vi "main.vi"() -> ()   [LabVIEW 2023]
panel:
  in  "Pause Game":bool
  in  "Decrease\nPlayer Length":bool
  in  "Stop":bool
  out "p2 score":i32
  out "p1 score":i32
  in  "w_bool":bool
  in  "Down_bool":bool
  in  "s_bool":bool
  in  "Up_bool":bool
  out "game window":picture
  # "Player 1: W, S\nPlayer 2: Up, Down"
  # "Modifiers"
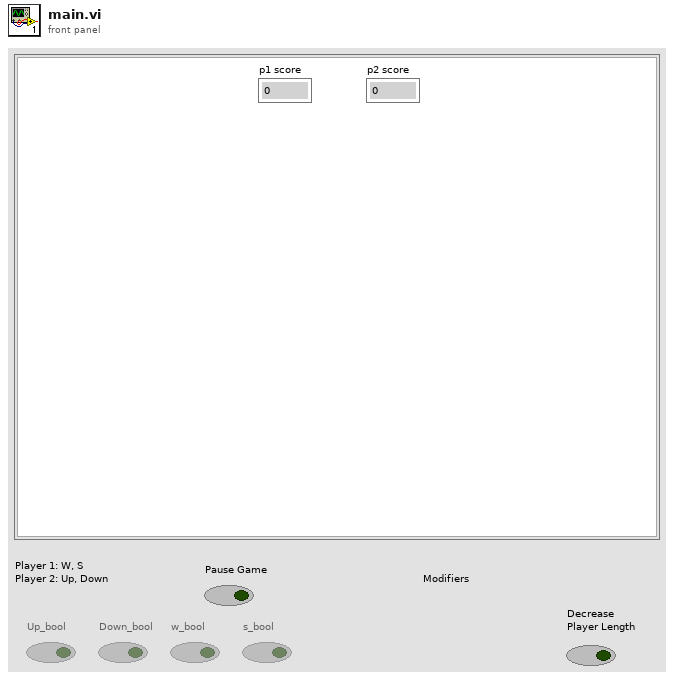
[diagram p1: front panel]
types:
  T1 = cluster{"output vector x":dbl, "output vector y":dbl}
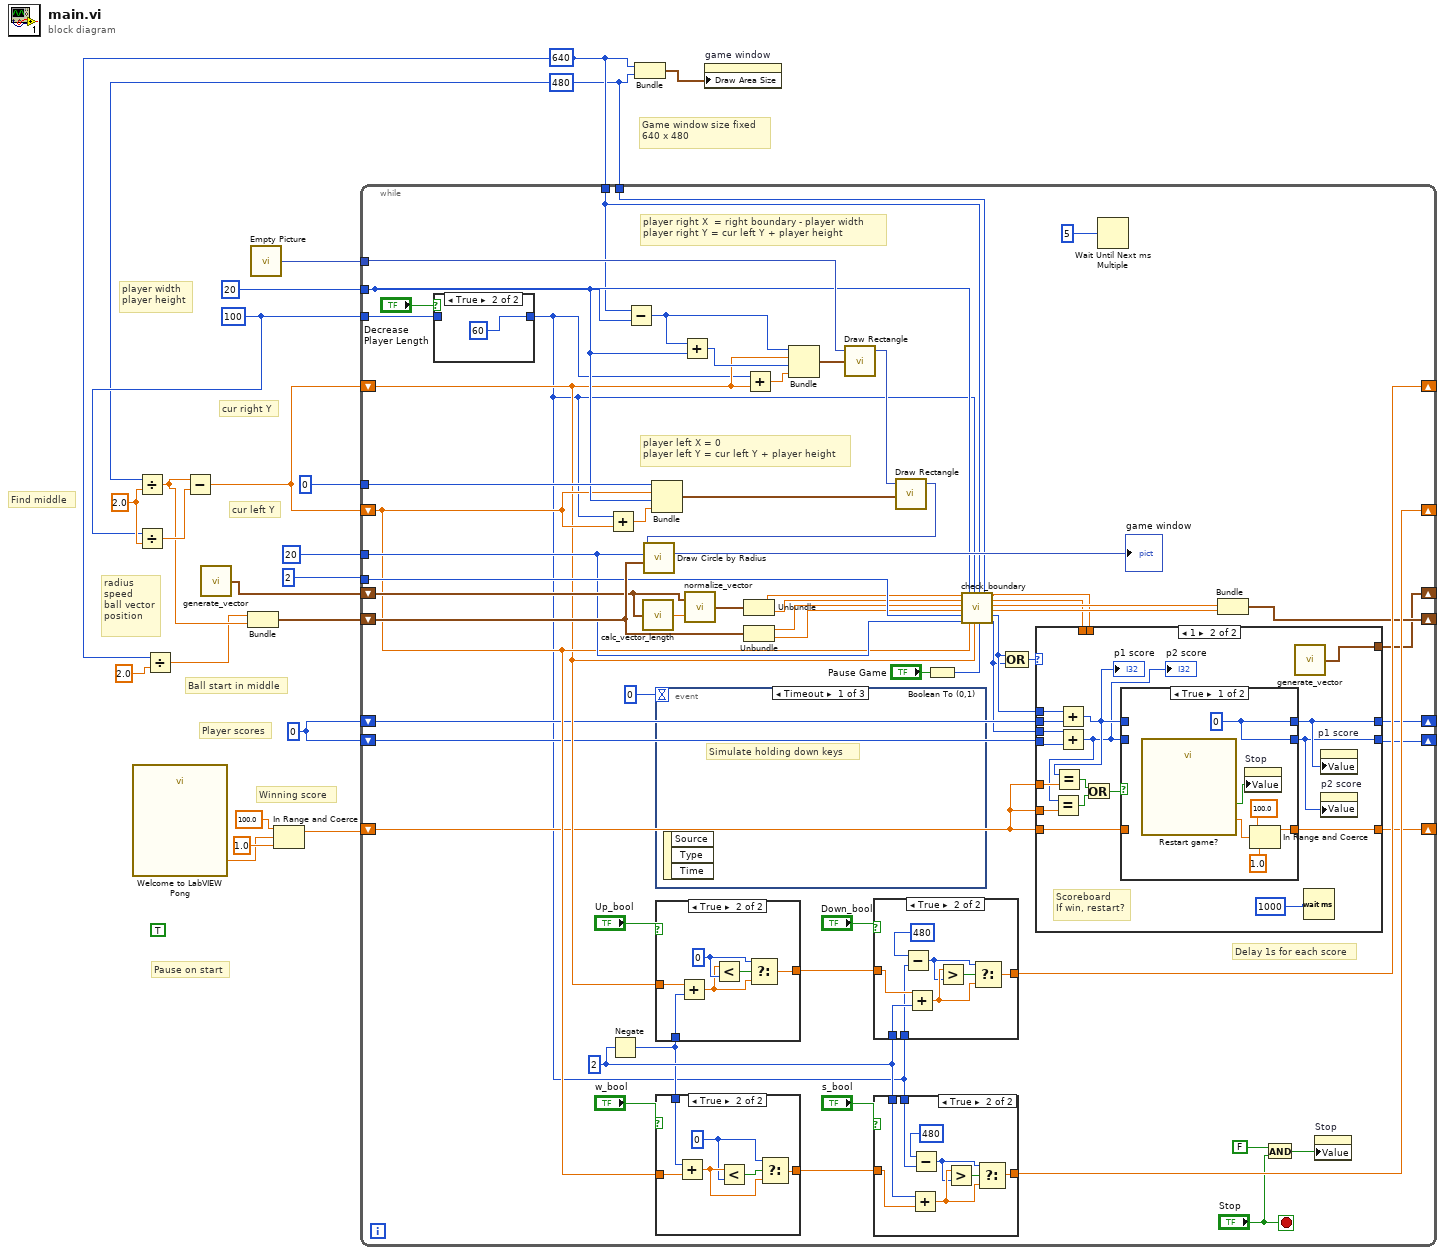
[diagram p0: block diagram]
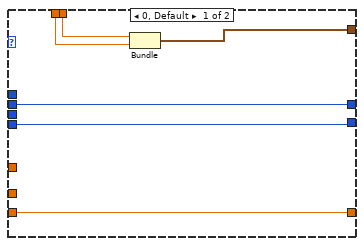
[diagram p3: hidden frame]
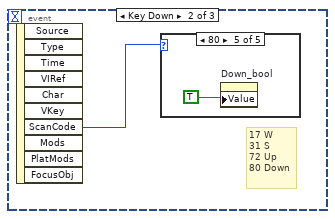
[diagram p9: hidden frame]
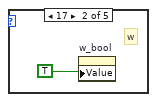
[diagram p11: hidden frame]
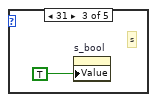
[diagram p12: hidden frame]
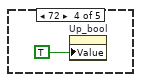
[diagram p13: hidden frame]
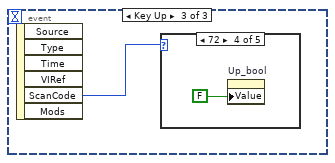
[diagram p14: hidden frame]
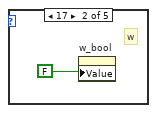
[diagram p16: hidden frame]
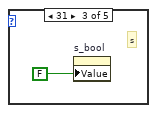
[diagram p17: hidden frame]
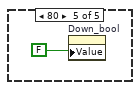
[diagram p18: hidden frame]
diagram:
  (unwired) TRUE ("Pause Game")
  w6 = 0
  w7 = 480
  w14 = 640
  w17 = 2.0 ("y")
  w15 = 100
  # "Pause on start"
  # "Winning score"
  # "Player scores"
  # "Ball start in middle"
  # "radius\nspeed\nball vector\nposition"
  # "Find middle"
  # "player width\nplayer height"
  # "cur left Y"
  # "cur right Y"
  # "Game window size fixed\n640 x 480"
  n1 = call "Welcome to LabVIEW Pong"() -> ("Winning Score"=w2:dbl)  [unwired: 17 in, 2 out]
  n2 = Divide(x=w7, y=w17) -> (x/y=w11:dbl)
  n3 = Divide(x=w15, y=w17) -> (x/y=w16:dbl)
  n4 = Divide(x=w14, y=2.0) -> (x/y=w10:dbl)
  n5 = Subtract(x=w11, y=w16) -> (x-y=w18:dbl)
  n6 = call "generate_vector.vi"() -> ("Cluster"=w5:cluster{"number":dbl, "number":dbl})
  n7 = Bundle(w10, w11) -> (w12:cluster{dbl, dbl})  [unwired: 1 in]
  n8 = call "Empty Picture"() -> ("empty picture"=w21:picture)
  n9 = In Range and Coerce(upper limit=100.0, x=w2, lower limit=1.0) -> (coerced(x)=w3:dbl)  [unwired: 1 out]
  n10 = while {
    tunnel: w14 -> [w50]
    tunnel: w21 -> [w80]
    shift-right: [w68] -> _
    shift-left: w18 -> [w43]
    shift-right: [w66] -> _
    shift-left: w18 -> [w44]
    tunnel: w15 -> [w27]
    tunnel: 20 -> [w51]
    tunnel: 0 -> [w78]
    shift-right: [w35] -> _
    shift-left: w5 -> [w57]
    shift-right: [w46] -> _
    shift-left: w12 -> [w60]
    tunnel: 20 -> [w45]
    tunnel: 2 -> [w56]
    tunnel: w7 -> [w49]
    shift-right: [w42] -> _
    shift-left: w6 -> [w40]
    shift-right: [w41] -> _
    shift-left: w6 -> [w39]
    shift-right: [w38] -> _
    shift-left: w3 -> [w31]
    stop <- "Stop" stop-if-true
    w71 = 2 ("y")
    # "Delay 1s for each score"
    # "player right X  = right boundary - player width\nplayer right Y = cur left Y + player height"
    # "player left X = 0\nplayer left Y = cur left Y + player height"
    n11 = case shown="True" "Decrease\nPlayer Length" {
      tunnel: w27 -> [w84 _]
      tunnel: [w84 60] -> w26
      frame False {
      }
      frame True {
      }
    }
    n12 = Add(x=w26, y=w44) -> (x+y=w77:dbl)
    n13 = Negate(x=w71) -> (-x=w70:i32)
    n14 = Subtract(x=w50, y=w51) -> (x-y=w83:i32)
    n15 = call "calc_vector_length.vi"("vector"=w57) -> ("length"=w58:dbl)
    n16 = Bundle(w78, w44, w51, w77) -> (w76:cluster{i32, dbl, i32, dbl})  [unwired: 1 in]
    n17 = event shown="[0] Timeout" {
      selector: _ -> [_ _ _]
      dyn-events: _ -> [_ _ _]
      timeout: 0 -> [_ _ _]
      event Timeout {
        # "Simulate holding down keys"
        n18 = event-data() -> ()  [unwired: 1 in, 3 out]
      }
      event Key Down {
        # "17 W\n31 S\n72 Up\n80 Down"
        n19 = event-data() -> ("ScanCode"=w150:i16)  [unwired: 1 in, 9 out]
        n20 = case shown="80" w150 {
          frame 0, Default {
          }
          frame 17 {
            # "w"
            n21 = property on="w_bool" class="Bool (strict)"("Value"=TRUE) -> ()  [unwired: 2 in, 2 out]
          }
          frame 31 {
            # "s"
            n22 = property on="s_bool" class="Bool (strict)"("Value"=TRUE) -> ()  [unwired: 2 in, 2 out]
          }
          frame 72 {
            n23 = property on="Up_bool" class="Bool (strict)"("Value"=TRUE) -> ()  [unwired: 2 in, 2 out]
          }
          frame 80 {
            n24 = property on="Down_bool" class="Bool (strict)"("Value"=TRUE) -> ()  [unwired: 2 in, 2 out]
          }
        }
      }
      event Key Up {
        n25 = event-data() -> ("ScanCode"=w155:i16)  [unwired: 1 in, 5 out]
        n26 = case shown="72" w155 {
          frame 0, Default {
          }
          frame 17 {
            # "w"
            n27 = property on="w_bool" class="Bool (strict)"("Value"=FALSE) -> ()  [unwired: 2 in, 2 out]
          }
          frame 31 {
            # "s"
            n28 = property on="s_bool" class="Bool (strict)"("Value"=FALSE) -> ()  [unwired: 2 in, 2 out]
          }
          frame 72 {
            n29 = property on="Up_bool" class="Bool (strict)"("Value"=FALSE) -> ()  [unwired: 2 in, 2 out]
          }
          frame 80 {
            n30 = property on="Down_bool" class="Bool (strict)"("Value"=FALSE) -> ()  [unwired: 2 in, 2 out]
          }
        }
      }
    }
    n31 = case shown="True" "Up_bool" {
      tunnel: w70 -> [_ w145]
      tunnel: w43 -> [w143 w146]
      tunnel: [w143 w144] -> w69
      frame False {
      }
      frame True {
        w148 = 0 ("y")
        n32 = Add(x=w146, y=w145) -> (x+y=w147:dbl)
        n33 = Less?(x=w147, y=w148) -> (x < y?=w149:bool)
        n34 = Select(t=w148, s=w149, f=w147) -> (s? t:f=w144:dbl)
      }
    }
    n35 = case shown="True" "w_bool" {
      tunnel: w44 -> [w136 w138]
      tunnel: w70 -> [_ w139]
      tunnel: [w136 w137] -> w67
      frame False {
      }
      frame True {
        w140 = 0 ("y")
        n36 = Add(x=w139, y=w138) -> (x+y=w142:dbl)
        n37 = Less?(x=w142, y=w140) -> (x < y?=w141:bool)
        n38 = Select(t=w140, s=w141, f=w142) -> (s? t:f=w137:dbl)
      }
    }
    n39 = Add(x=w83, y=w51) -> (x+y=w82:i32)
    n40 = call "normalize_vector.vi"("Numeric"=w58, "vector"=w57) -> ("output"=w59:cluster{"x":dbl, "y":dbl})
    n41 = Unbundle(w59) -> ("x"=w55:dbl, "y"=w54:dbl)
    n42 = Unbundle(w60) -> (w53:dbl, w52:dbl)
    n43 = Add(x=w26, y=w43) -> (x+y=w81:dbl)
    n44 = Bundle(w83, w43, w82, w81) -> (w79:cluster{i32, dbl, i32, dbl})  [unwired: 1 in]
    n45 = call <vilib>:"Draw Rectangle.vi"("picture"=w80, "rect"=w79) -> ("new picture"=w75:picture)  [unwired: 7 in]
    n46 = case shown="True" "Down_bool" {
      tunnel: w71 -> [_ w131]
      tunnel: w69 -> [w127 w130]
      tunnel: [w127 w129] -> w68
      tunnel: w26 -> [_ w128]
      frame False {
      }
      frame True {
        n47 = Subtract(x=480 ("y"), y=w128) -> (x-y=w133:i32)
        n48 = Add(x=w130, y=w131) -> (x+y=w134:dbl)
        n49 = Greater?(x=w134, y=w133) -> (0:w135:bool)
        n50 = Select(t=w133, s=w135, f=w134) -> (s? t:f=w129:dbl)
      }
    }
    n51 = case shown="True" "s_bool" {
      tunnel: w71 -> [_ w121]
      tunnel: w67 -> [w118 w122]
      tunnel: [w118 w120] -> w66
      tunnel: w26 -> [_ w119]
      frame False {
      }
      frame True {
        n52 = Add(x=w121, y=w122) -> (x+y=w125:dbl)
        n53 = Subtract(x=480 ("y"), y=w119) -> (x-y=w124:i32)
        n54 = Greater?(x=w125, y=w124) -> (0:w126:bool)
        n55 = Select(t=w124, s=w126, f=w125) -> (s? t:f=w120:dbl)
      }
    }
    n56 = call <vilib>:"Draw Rectangle.vi"("picture"=w75, "rect"=w76) -> ("new picture"=w62:picture)  [unwired: 7 in]
    n57 = call <vilib>:"Draw Circle by Radius.vi"("pixel center"=w60, "radius"=w45, "picture"=w62) -> ("new picture"=→"game window":picture)  [unwired: 8 in]
    n58 = Boolean To (0,1)(Boolean="Pause Game") -> (0, 1=w23:i16)
    n59 = call "check_boundary.vi"("vector x"=w55, "vector y"=w54, "position x"=w53, "position y"=w52, "speed"=w56, "radius"=w45, "player width"=w51, "player left position y"=w44, "player height"=w26, "player right position y"=w43, "window width"=w50, "pause"=w23, "window height"=w49) -> ("output vector x"=w37:dbl, "output vector y"=w36:dbl, "output x"=w48:dbl, "output y"=w47:dbl, "left win"=w29:i32, "right win"=w28:i32)  [unwired: 1 in]
    n60 = Compound Arithmetic op=OR(w29, w28) -> (w30:i32)
    n61 = case shown="1" w30 {
      tunnel: w40 -> [w91 w99]
      tunnel: w39 -> [w90 w97]
      tunnel: w29 -> [_ w100]
      tunnel: w28 -> [_ w98]
      tunnel: [w91 w93] -> w42
      tunnel: [w90 w92] -> w41
      tunnel: w31 -> [_ w108]
      tunnel: w31 -> [_ w107]
      tunnel: [w89 w103] -> w38
      tunnel: w31 -> [w89 w102]
      tunnel: w37 -> [w88 _]
      tunnel: w36 -> [w87 _]
      tunnel: [w86 w101] -> w35
      frame 0, Default {
        n62 = Bundle("output vector x"=w88, "output vector y"=w87) -> (w86:T1)  [unwired: 1 in]
      }
      frame 1 {
        # "Scoreboard\nIf win, restart?"
        n63 = Add(x=w100, y=w99) -> (x+y=w95:i32)
        "p1 score" <- w95
        n64 = Equal?(x=w95, y=w108) -> (x = y?=w105:bool)
        n65 = Add(x=w98, y=w97) -> (x+y=w94:i32)
        "p2 score" <- w94
        n66 = Equal?(x=w94, y=w107) -> (x = y?=w104:bool)
        n67 = Or(x=w105, y=w104) -> (x .or. y?=w106:bool)
        n68 = case shown="True" w106 {
          tunnel: [w113 w115] -> w92
          tunnel: [w113 w116] -> w93
          tunnel: [w110 w117] -> w103
          tunnel: w102 -> [_ w117]
          tunnel: w95 -> [_ w116]
          tunnel: w94 -> [_ w115]
          frame True {
            w113 = 0
            n69 = call "Restart game?"() -> ("Winning Score"=w109:dbl, "Quit game"=w114:bool)  [unwired: 17 in, 1 out]
            n70 = property on="Stop" class="Bool (strict)"("Value"=w114) -> ()  [unwired: 2 in, 2 out]
            n71 = In Range and Coerce(upper limit=100.0, x=w109, lower limit=1.0) -> (coerced(x)=w110:dbl)  [unwired: 1 out]
          }
          frame False {
          }
        }
        n72 = call "generate_vector.vi"() -> ("Cluster"=w101:cluster{"number":dbl, "number":dbl})
        n73 = Wait (ms)(milliseconds to wait=u32 1000) -> ()  [unwired: 1 out]
        n74 = property on="p1 score" class="DigNum (strict)"("Value"=w93) -> ()  [unwired: 2 in, 2 out]
        n75 = property on="p2 score" class="DigNum (strict)"("Value"=w92) -> ()  [unwired: 2 in, 2 out]
      }
    }
    n76 = Wait Until Next ms Multiple(millisecond multiple=u32 5 ("milliseconds to wait")) -> ()  [unwired: 1 out]
    n77 = Bundle("output x"=w48, "output y"=w47) -> (w46:cluster{"output x":dbl, "output y":dbl})  [unwired: 1 in]
    n78 = And(x=FALSE, y="Stop") -> (x .and. y?=w32:bool)
    n79 = property on="Stop" class="Bool (strict)"("Value"=w32) -> ()  [unwired: 2 in, 2 out]
  }
  n80 = Bundle(w14, w7) -> (w22:cluster{i32, i32})  [unwired: 1 in]
  n81 = property on="game window" class="Pict"("Draw Area Size"=w22) -> ()  [unwired: 2 in, 2 out]
